vi "Test - Explain Better Error.vi"() -> ()   [LabVIEW 2020]
panel:
  out "error in (no error)":errorcluster={"status"=FALSE, "code"=7, "source"=""}
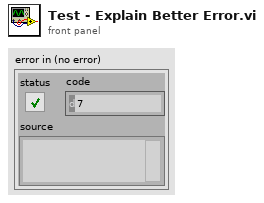
[diagram p1: front panel]
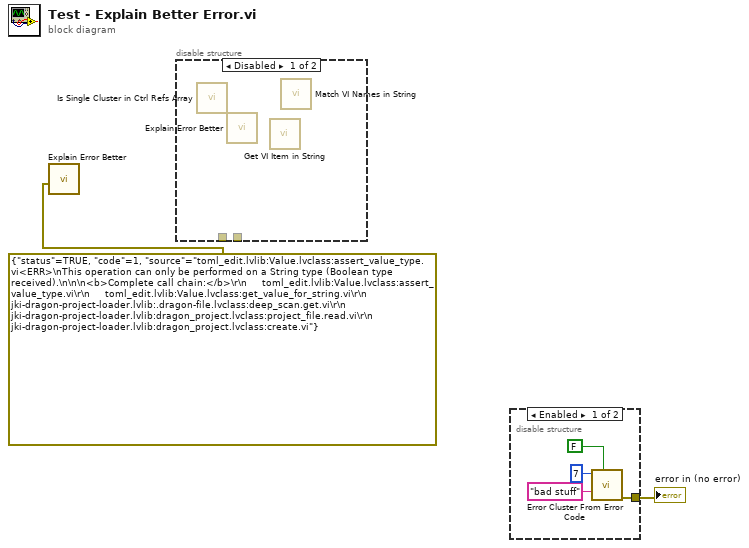
[diagram p0: block diagram]
diagram:
  n1 = call <resource>:"Explain Error Better.vi"("Error Cluster"=errorcluster {"status"=TRUE, "code"=1, "source"="toml_edit.lvlib:Value.lvclass:assert_value_type.vi<ERR>\nThis operation can only be performed on a String type (Boolean type received).\n\n\n<b>Complete call chain:</b>\r\n     toml_edit.lvlib:Value.lvclass:assert_value_type.vi\r\n     toml_edit.lvlib:Value.lvclass:get_value_for_string.vi\r\n     jki-dragon-project-loader.lvlib:.dragon-file.lvclass:deep_scan.get.vi\r\n     jki-dragon-project-loader.lvlib:dragon_project.lvclass:project_file.read.vi\r\n     jki-dragon-project-loader.lvlib:dragon_project.lvclass:create.vi"}) -> ()  [unwired: 11 in]
  n2 = disable-structure shown="Disabled" {
    disable-tunnel: _ -> [w4 _]
    disable-tunnel: _ -> [w3 _]
    frame Disabled {
      n3 = call <resource>:"Is Single Cluster in Ctrl Refs Array.vi"() -> ()  [unwired: 10 in, 2 out]
      n4 = call <resource>:"Explain Error Better.vi"() -> ()  [unwired: 12 in]
      n5 = call <resource>:"Get VI Item in String.vi"() -> ()  [unwired: 8 in, 4 out]
      n6 = call <resource>:"Match VI Names in String.vi"() -> ()  [unwired: 11 in, 1 out]
    }
    frame Enabled {
    }
  }
  n7 = disable-structure shown="Enabled" {
    disable-tunnel: [w8 _] -> w2
    frame Enabled {
      n8 = call <vilib>:"Error Cluster From Error Code.vi"("show call chain? (False)"=FALSE, "error message (\"\")"="bad stuff" ("error message (\"\")"), "error code (0)"=7) -> ("error out"=w8:errorcluster)  [unwired: 6 in]
    }
    frame Disabled {
    }
  }
  "error in (no error)" <- w2
